vi "Product and Serial number details.vi"(8 "Error In":errorcluster) -> (0 "Error Out":errorcluster, 3 "Product and Serial Number":string[][](array[string]))   [LabVIEW 2010]
uses:
  <vilib>/nisyscfg/Find Hardware.vi
  <vilib>/nisyscfg/Close (System).vi
  <vilib>/nisyscfg/Close (Hardware).vi
  <vilib>/nisyscfg/nisyscfg.lvlib
  Program Files/National Instruments/LabVIEW 2010/resource/objmgr/nisysapi.rc
panel:
  in  "Actual Results from Hardware":string[][](array[string])=[["NI PXI-2530", "0165D6B5", "{3B009CCE-19F3-11E1-80D0-A31CDBA49E0A}", "PXI3Slot5"], ["NI PXI-2532", "00ECDC25", "{40CDF5D4-19F3-11E1-80D0-A31CDBA49E0A}", "PXI3Slot6"], ["NI PXI-2568", "", "{5C7D2836-3AF0-11E1-8067-B38294519752}", "PXI4Slot2"], ["NI PXI-6509", "0163D45F", "{A6BB28FC-00CC-11E1-804A-826C7DE95087}", "PXI2Slot3"], ["NI PXI-5122", "00F05AAD", "{ADA439D8-00CC-11E1-804A-826C7DE95087}", "PXI1Slot4"], ["NI PXI-2532", "00EDFE22", "{B48BA078-0000-11E1-80CF-930EF23638A5}", "PXI2Slot6"], ["NI PXI-2530", "0155AEAE", "{BDCB1F92-0000-11E1-80CF-930EF23638A5}", "PXI2Slot5"], ["NI PXI-2530", "0155AEAC", "{C7358900-0000-11E1-80CF-930EF23638A5}", "PXI2Slot4"], ["NI PXI-5122", "00EE9092", "{CDA29F94-0000-11E1-80CF-930EF23638A5}", "PXI1Slot6"], ["PCI-GPIB", "01617EC4", "c000006f", ""], ["", "", "c0000033", ""], ["", "", "c0000037", ""], ["", "", "c000003b", ""], ["NI PXI-1033", "", "PXICHASSIS1", "Chassis 1"], ["NI PXI-1033", "", "PXICHASSIS2", "Chassis 2"], ["NI PXI-1033", "", "PXICHASSIS3", "Chassis 3"], ["4040A", "", "PXI4::12::INSTR", ""], ["Geotest GTX2200 High Resolution Universal Time Interval Counter Board", "", "PXI4::15::INSTR", ""], ["4040A", "", "PXI4::14::INSTR", ""], ["", "", "ASRL1::INSTR", "COM1"], ["", "", "ASRL10::INSTR", "LPT1"], ["", "", "GPIB0::7::INSTR", ""], ["", "", "GPIB0::6::INSTR", ""], ["", "", "GPIB0::8::INSTR", ""], ["", "", "GPIB0::9::INSTR", ""], ["", "", "GPIB0::10::INSTR", ""]]
  # "Agilent Technologies,33210A,MY48005963,1.04-1.04-22-2"
  # "KEITHLEY INSTRUMENTS INC.,MODEL 2400,1308532,C32   Oct  4 2010 14:20:11/A02  /R/J"
  # "KEITHLEY INSTRUMENTS INC.,MODEL 2000,1308410,A20  /A02"
  # "KEITHLEY INSTRUMENTS INC.,MODEL 2400,1308737,C32   Oct  4 2010 14:20:11/A02  /R/J"
  # "KEITHLEY INSTRUMENTS INC.,MODEL 2400,1308731,C32   Oct  4 2010 14:20:11/A02  /R/J"
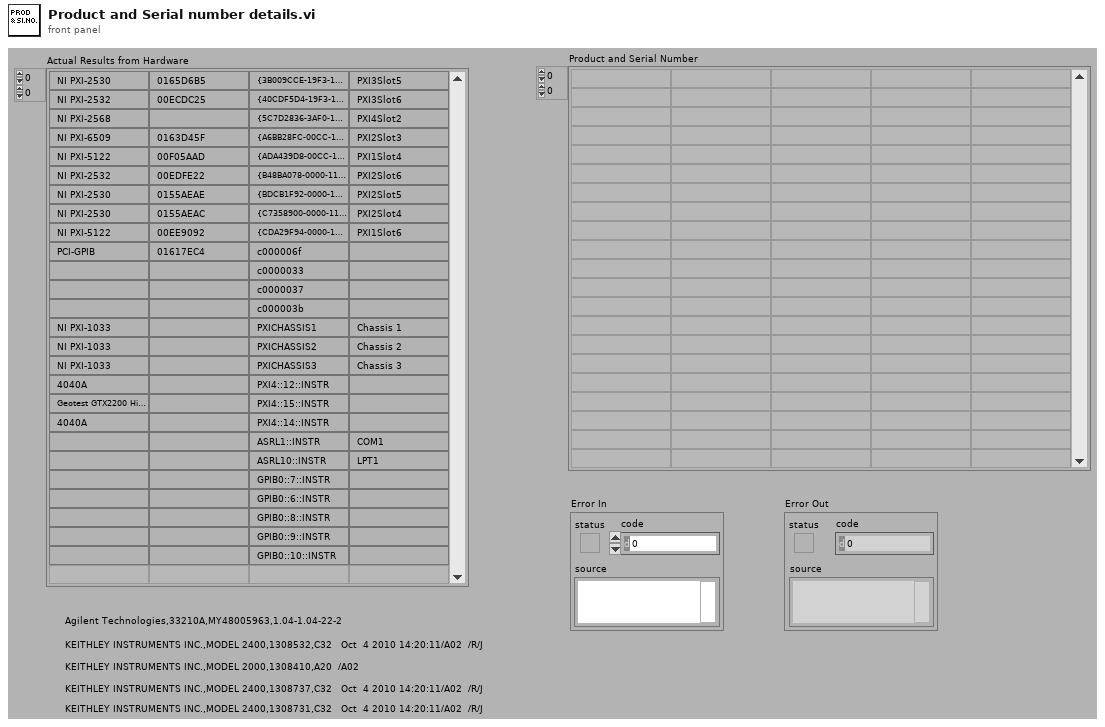
[diagram p1: front panel]
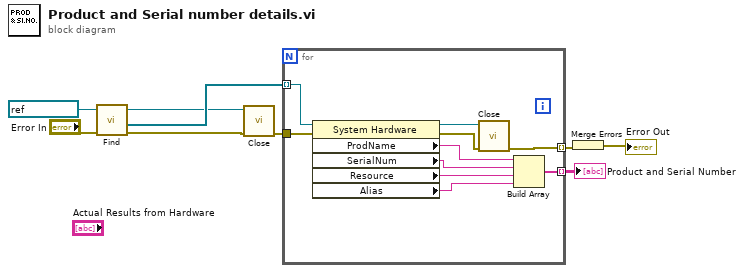
[diagram p0: block diagram]
diagram:
  n1 = call-poly <vilib>:"Find.vi"("error in (no error)"="Error In", "session in"=refnum<k21> "localhost") -> ("error out"=w6:errorcluster, "resources out"=w9:refnum<k20>[], "session out"=w7:refnum<k21>)  [unwired: 6 in, 1 out]
  n2 = call-poly <vilib>:"Close.vi"("error in (no error)"=w6, "session in"=w7) -> ("error out"=w5:errorcluster)  [unwired: 9 in]
  n3 = for {
    tunnel: w9 -> [w19] mode=indexing
    tunnel: w5 -> [w18]
    tunnel: [w15] -> w2 mode=indexing
    tunnel: [w12] -> w4 mode=indexing
    n4 = property class="System Hardware"(reference=w19, error in=w18) -> (reference out=w17:refnum<k20>, error out=w16:errorcluster, "ProdName"=w14:string, "SerialNum"=w13:string, "Resource"=w11:string, "Alias"=w10:string)
    n5 = call-poly <vilib>:"Close.vi"("error in (no error)"=w16, "resource in"=w17) -> ("error out"=w15:errorcluster)  [unwired: 9 in]
    n6 = Build Array(w14, w13, w11, w10) -> (w12:string[])
  }
  "Product and Serial Number" <- w4
  n7 = Merge Errors(w2) -> (→"Error Out":errorcluster)
